vi "find_repeat_parameters_1.vi"(8 "error in (no error)":errorcluster, 11 "String In":string="SENSe[1]|SENSe2:SWEep[1]|2|3|4:TIME <numeric_value>") -> (0 "error out":errorcluster, 3 "String Out":string="SENSe{<n>}:SWEep[1]|2|3|4:TIME <numeric_value>")   [LabVIEW 2018]
uses:
  <vilib>/regexp/Match Regular Expression.xnode
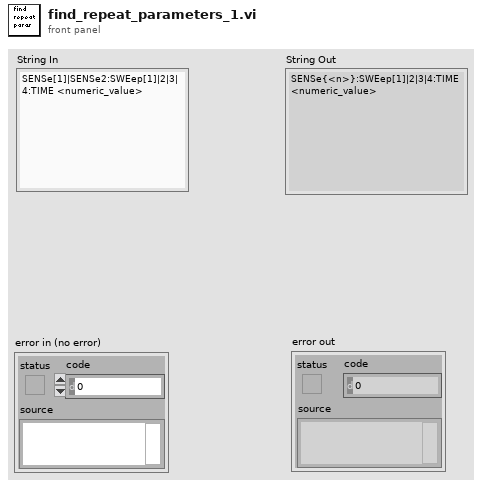
[diagram p1: front panel]
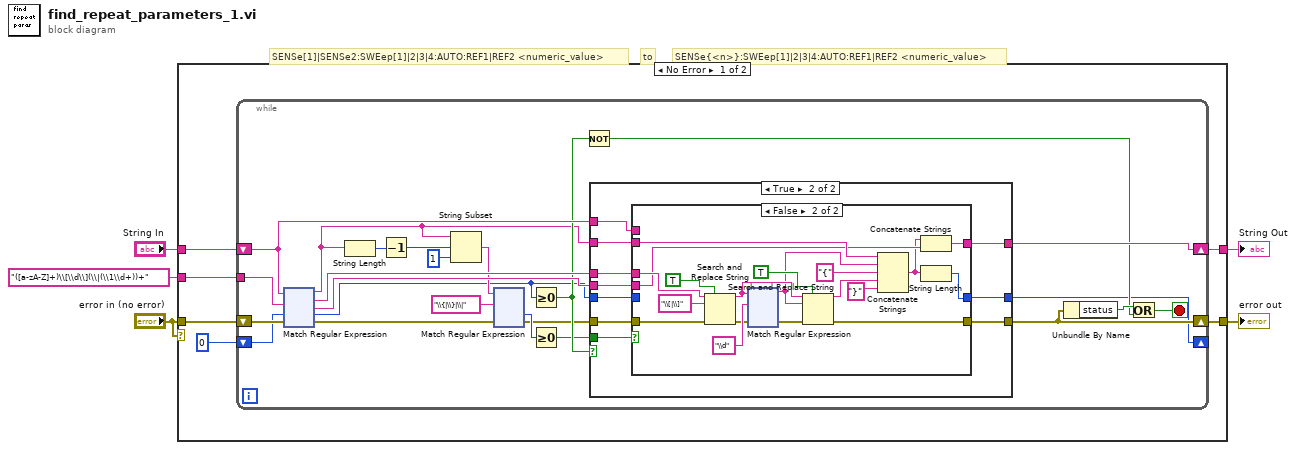
[diagram p0: block diagram]
diagram:
  # "to"
  # "SENSe{<n>}:SWEep[1]|2|3|4:AUTO:REF1|REF2 <numeric_value>"
  # "SENSe[1]|SENSe2:SWEep[1]|2|3|4:AUTO:REF1|REF2 <numeric_value>"
  n1 = case shown="No Error" "error in (no error)" {
    tunnel: "([a-zA-Z]+)\\[\\d\\](\\|(\\1\\d+))+" ("regular expression") -> [w11 _]
    tunnel: "String In" -> [w10 w405]
    tunnel: "error in (no error)" -> [w9 w404]
    tunnel: [w8 w405] -> w3
    tunnel: [w7 w404] -> w2
    frame No Error {
      n2 = while {
        tunnel: w11 -> [w35]
        shift-right: [w31] -> w8
        shift-left: w10 -> [w33]
        shift-right: [w25] -> w7
        shift-left: w9 -> [w32]
        shift-right: [w13] -> _
        shift-left: 0 -> [w16]
        stop <- w26 stop-if-true
        n3 = xnode "Match Regular Expression"("input string"=w33, "regular expression"=w35, "offset (0)"=w16, "error in"=w32) -> ("before match"=w15:string, "whole match"=w34:string, "after match"=w30:string, "offset past match"=w12:i32, "error out"=w18:errorcluster)  [unwired: 2 out]
        n4 = String Length(string=w15) -> (length=w21:i32)
        n5 = Decrement(x=w21) -> (x-1=w20:i32)
        n6 = String Subset(string=w15, offset (0)=w20, length (rest)=1 ("length (rest)")) -> (substring=w23:string)
        n7 = xnode "Match Regular Expression"("input string"=w23, "regular expression"="\\{|\\}|\\|", "error in"=w18) -> ("offset past match"=w19:i32, "error out"=w17:errorcluster)  [unwired: 1 in, 5 out]
        n8 = Greater Or Equal To 0?(x=w12) -> (x >= 0?=w29:bool)
        n9 = Greater Or Equal To 0?(x=w19) -> (x >= 0?=w14:bool)
        n10 = Not(x=w29) -> (.not. x?=w27:bool)
        n11 = case shown="True" w29 {
          tunnel: w34 -> [_ w48]
          tunnel: w33 -> [w38 w43]
          tunnel: [w38 w47] -> w31
          tunnel: w17 -> [w37 w42]
          tunnel: [w37 w41] -> w25
          tunnel: w15 -> [_ w46]
          tunnel: w30 -> [_ w45]
          tunnel: w14 -> [_ w44]
          tunnel: [w36 w40] -> w13
          tunnel: w12 -> [w36 w39]
          frame False {
          }
          frame True {
            n12 = case shown="False" w44 {
              tunnel: w48 -> [_ w60]
              tunnel: [w51 w54] -> w47
              tunnel: w46 -> [_ w68]
              tunnel: w45 -> [_ w55]
              tunnel: w43 -> [w51 _]
              tunnel: w42 -> [w50 w59]
              tunnel: [w50 w56] -> w41
              tunnel: [w49 w52] -> w40
              tunnel: w39 -> [w49 _]
              frame True {
              }
              frame False {
                n13 = Search and Replace String(replace all?=TRUE ("replace all? (F)"), input string=w60, search string="\\[|\\]", error in=w59) -> (result string=w65:string, error out=w58:errorcluster)  [unwired: 6 out]
                n14 = xnode "Match Regular Expression"("input string"=w65, "regular expression"="\\d", "error in"=w58) -> ("before match"=w64:string, "error out"=w57:errorcluster)  [unwired: 1 in, 5 out]
                n15 = Search and Replace String(replace all?=TRUE ("replace all? (F)"), input string=w65, search string=w64, error in=w57) -> (result string=w63:string, error out=w56:errorcluster)  [unwired: 6 out]
                n16 = Concatenate Strings(w68, w64, "{" ("string"), w63, "}" ("string")) -> (w53:string)
                n17 = Concatenate Strings(w53, w55) -> (w54:string)
                n18 = String Length(string=w53) -> (length=w52:i32)
              }
            }
          }
        }
        n19 = Unbundle By Name(w25) -> ("status"=w28:bool)
        n20 = Or(x=w28, y=w27) -> (x .or. y?=w26:bool)
      }
    }
    frame Error {
    }
  }
  "String Out" <- w3
  "error out" <- w2
